vi "Read Caller Enqueuer.vi"(8 "error in (no error)":errorcluster, 11 "Replay Msg in":refnum<class "Replay Msg.lvclass">) -> (0 "error out":errorcluster, 2 "Enqueuer":refnum<class "Message Enqueuer.lvclass">, 3 "Replay Msg out":refnum<class "Replay Msg.lvclass">)   [LabVIEW 2014, in "Replay Msg.lvclass"]
uses:
  ExperimentService/Replay Msg.lvclass
  <vilib>/ActorFramework/Message Enqueuer/Message Enqueuer.lvclass
  ExperimentService/Replay Msg.lvclass/Replay Msg.ctl
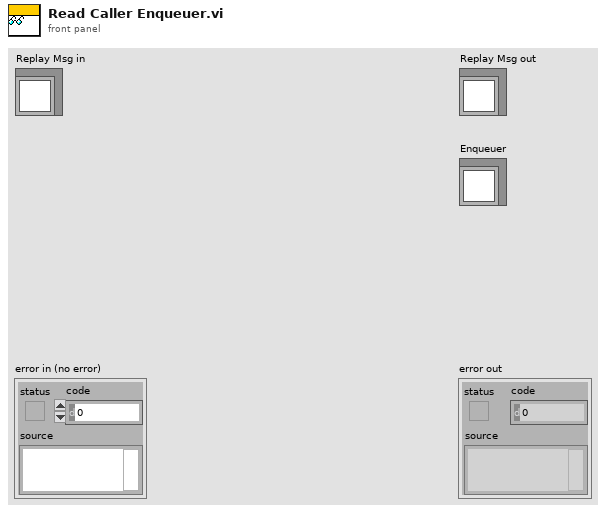
[diagram p1: front panel]
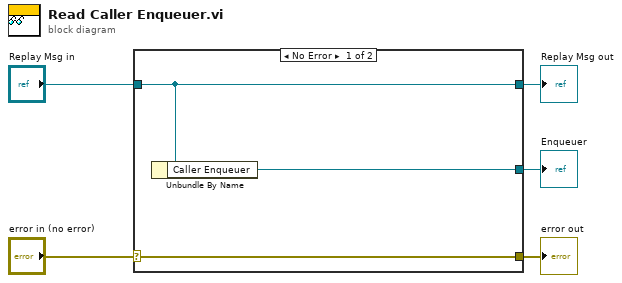
[diagram p0: block diagram]
diagram:
  n1 = case shown="No Error" "error in (no error)" {
    selector: "error in (no error)" -> [w8 w9]
    tunnel: [w8 w9] -> w4
    tunnel: [w7 w10] -> w2
    tunnel: "Replay Msg in" -> [w7 w10]
    tunnel: [w6 _] -> w1
    frame No Error {
      n2 = Unbundle By Name(w7) -> ("Caller Enqueuer"=w6:refnum<class "Message Enqueuer.lvclass">)
    }
    frame Error {
    }
  }
  "error out" <- w4
  "Replay Msg out" <- w2
  "Enqueuer" <- w1
